vi "Transfer File.vi"(8 "error in (no error)":errorcluster) -> (0 "error out":errorcluster)   [LabVIEW 2017]
uses:
  <vilib>/WebDAVClient/NI_WebDAV.lvlib
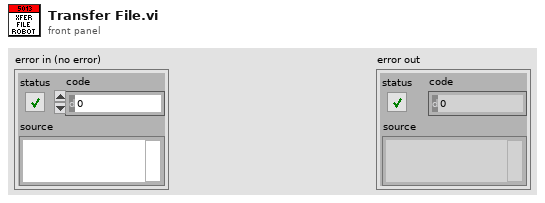
[diagram p1: front panel]
types:
  T1 = typedef "NI_WebDAV.lvlib/SessionHandle.ctl" = refnum<k1>
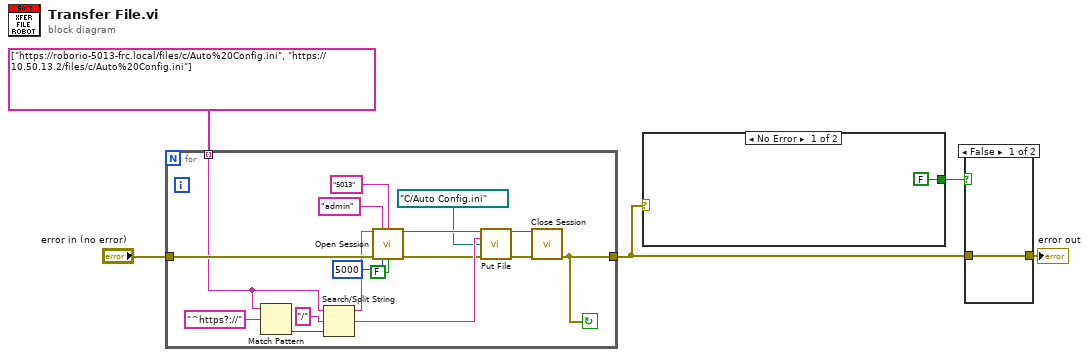
[diagram p0: block diagram]
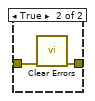
[diagram p2: hidden frame]
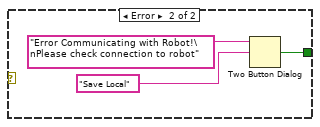
[diagram p3: hidden frame]
diagram:
  n1 = for {
    tunnel: string[] ["https://roborio-5013-frc.local/files/c/Auto%20Config.ini", "https://10.50.13.2/files/c/Auto%20Config.ini"] ("file uri") -> [w15] mode=indexing
    tunnel: "error in (no error)" -> [w22]
    tunnel: [w7] -> w3
    stop <- w7 continue-if-true
    n2 = Match Pattern(string=w15, regular expression="^https?://") -> (offset past match=w21:i32)  [unwired: 1 in, 3 out]
    n3 = Search/Split String(string=w15, search string/char (-)="/", offset (0)=w21) -> (substring before match=w18:string, match + rest of string=w10:string)  [unwired: 1 out]
    n4 = call <vilib>:"Open Session.vi"("host uri prefix"=w18, "username"="admin", "password"="5013", "error in (no error)"=w22, "timeout ms"=5000, "verify server?"=FALSE) -> ("session handle out"=w11:T1, "error out"=w9:errorcluster)  [unwired: 8 in]
    n5 = call <vilib>:"Put File.vi"("session handle"=w11, "relative uri"=w10, "local file path"=path "C:/Auto Config.ini" ("Path (dialog)"), "error in (no error)"=w9) -> ("session handle out"=w13:T1, "error out"=w12:errorcluster)  [unwired: 9 in, 1 out]
    n6 = call <vilib>:"Close Session.vi"("session handle"=w13, "error in (no error)"=w12) -> ("error out"=w7:errorcluster)  [unwired: 13 in]
  }
  n7 = case shown="No Error" w3 {
    tunnel: [FALSE ("T button?") w24] -> w2
    frame No Error {
    }
    frame Error {
      n8 = Two Button Dialog(message="Error Communicating with Robot!\nPlease check connection to robot", 2:"Save Local" ("T button name (\"OK\")")) -> (T button?=w24:bool)  [unwired: 1 in]
    }
  }
  n9 = case shown="False" w2 {
    tunnel: w3 -> [w27 w29]
    tunnel: [w27 w28] -> w1
    frame False {
    }
    frame True {
      n10 = call <vilib>:"Clear Errors.vi"("error in (no error)"=w29) -> ("error out"=w28:errorcluster)  [unwired: 5 in, 1 out]
    }
  }
  "error out" <- w1
